vi "sta_Covarance Matrix(SubVI).vi"(8 "에러 입력(에러 없음)":errorcluster, 11 "x":dbl[][](array[numeric])) -> (0 "에러 출력":errorcluster, 1 "mean vector":dbl[](array[numeric]) caption="평균 벡터", 2 "covariance matrix V":dbl[][](array[numeric]), 3 "참조 번호 출력":refnum<k35>)   [LabVIEW 2018]
uses:
  PythonConfigGlobal.vi
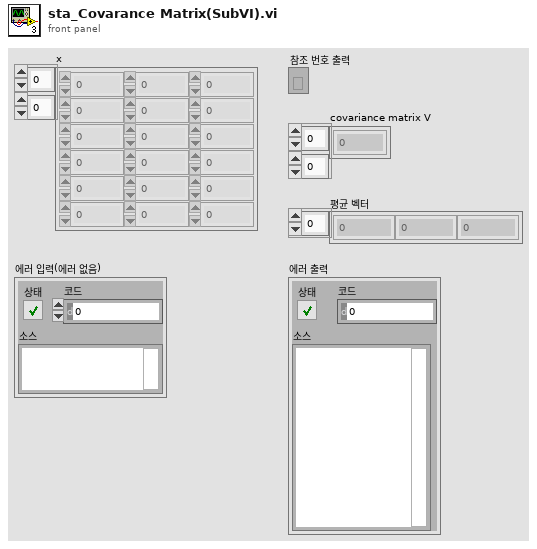
[diagram p1: front panel]
types:
  T1 = cluster{"covariance matrix V":dbl[][], "mean vector":dbl[]}
  T2 = cluster{"session out":refnum<k35>, "appended path":path}
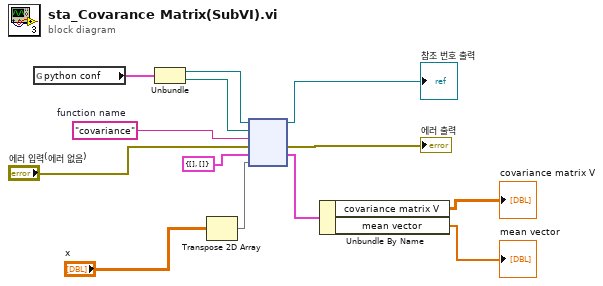
[diagram p0: block diagram]
diagram:
  w1 = "covariance"  # function name
  n1 = global read "PythonConfigGlobal.vi" "python conf"() -> (w6:T2)
  n2 = Unbundle(w6) -> ("session out"=w2:refnum<k35>, "appended path"=w3:path)
  n3 = Transpose 2D Array(2D array="x") -> (transposed array=w9:dbl[][])
  n4 = node(w2, w3, w1, "에러 입력(에러 없음)", T1 {"covariance matrix V"=[], "mean vector"=[]}, w9) -> (→"참조 번호 출력":refnum<k35>, →"에러 출력":errorcluster, w11:T1)  [unwired: 1 in, 2 out]
  n5 = Unbundle By Name(w11) -> ("covariance matrix V"=→"covariance matrix V":dbl[][], "mean vector"=→"mean vector":dbl[])
